vi "Postfix Stack.vi"(8 "error in (no error)":errorcluster, 10 "Variable Names":string[](array[string]), 11 "Postfix":T2[](array[typedef])) -> (0 "error out":errorcluster, 2 "Values":dbl[](array[numeric]), 3 "Types":T1[](array[typedef]))   [LabVIEW 2022 SP3, in "Expressions.lvlib"]
uses:
  Expressions.lvlib
  Controls/Token.ctl
  Controls/Token Type.ctl
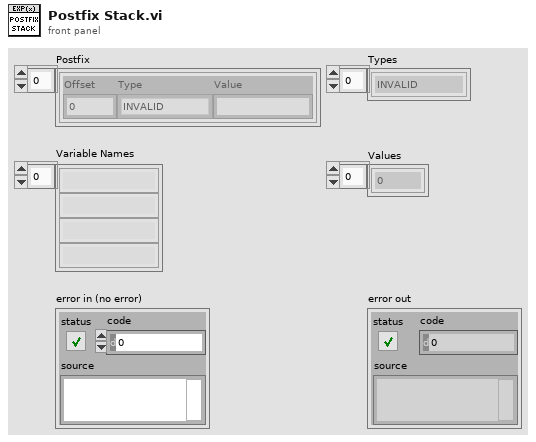
[diagram p1: front panel]
types:
  T1 = typedef "Expressions.lvlib/Token Type.ctl" = enum8{"INVALID", "NOT", "AND", "OR", "EE", "NE", "LT", "GT", "LTE", "GTE", "PLUS", "MINUS", "MULTIPLY", "DIVIDE", "MODULUS", "LPAREN", "RPAREN", "LITERAL", "IDENTIFIER", "DEFINITION"}
  T2 = typedef "Expressions.lvlib/Token.ctl" = cluster{"Offset":i32, "Type":T1, "Value":string}
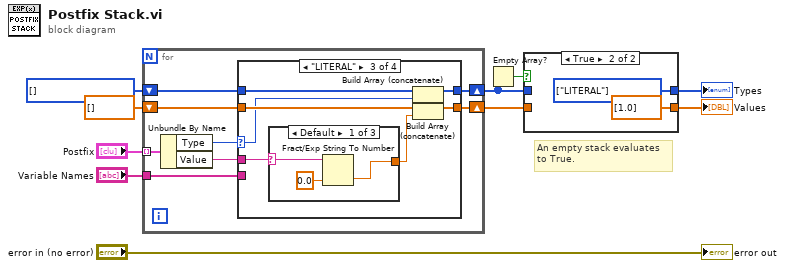
[diagram p0: block diagram]
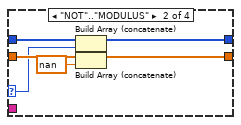
[diagram p4: hidden frame]
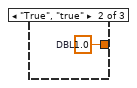
[diagram p5: hidden frame]
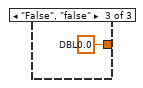
[diagram p6: hidden frame]
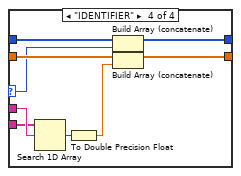
[diagram p7: hidden frame]
diagram:
  w9 = T1[] [] items=["INVALID", "NOT", "AND", "OR", "EE", "NE", "LT", "GT", "LTE", "GTE", "PLUS", "MINUS", "MULTIPLY", "DIVIDE", "MODULUS", "LPAREN", "RPAREN", "LITERAL", "IDENTIFIER", "DEFINITION"]
  # "An empty stack evaluates\nto True."
  n1 = for {
    tunnel: "Postfix" -> [w18] mode=indexing
    shift-right: [w16] -> w7
    shift-left: w9 -> [w15]
    shift-right: [w13] -> w5
    shift-left: dbl[] [] ("Values") -> [w14]
    tunnel: "Variable Names" -> [w11]
    n2 = Unbundle By Name(w18) -> ("Type"=w17:T1, "Value"=w12:string)
    n3 = case shown="\"LITERAL\"" w17 {
      selector: w17 -> [_ w22 w29 w43]
      tunnel: [w20 w24 w31 w45] -> w16
      tunnel: w15 -> [w20 w26 w33 w47]
      tunnel: w14 -> [w19 w25 w32 w46]
      tunnel: [w19 w23 w30 w44] -> w13
      tunnel: w12 -> [_ _ w28 w42]
      tunnel: w11 -> [_ _ _ w41]
      frame "INVALID", "LPAREN", "RPAREN", "DEFINITION" {
      }
      frame "NOT".."MODULUS" {
        n4 = Build Array (concatenate)(w26, w22) -> (w24:T1[])
        n5 = Build Array (concatenate)(w25, nan) -> (w23:dbl[])
      }
      frame "LITERAL" {
        n6 = case shown="Default" w28 {
          selector: w28 -> [w36 _ _]
          tunnel: [w34 w37 w38] -> w27
          frame Default {
            n7 = Fract/Exp String To Number(string=w36, default (0 dbl)=0.0 ("DBL")) -> (number=w34:dbl)  [unwired: 2 in, 1 out]
          }
          frame "True", "true" {
            w37 = 1.0  # DBL
          }
          frame "False", "false" {
            w38 = 0.0  # DBL
          }
        }
        n8 = Build Array (concatenate)(w33, w29) -> (w31:T1[])
        n9 = Build Array (concatenate)(w32, w27) -> (w30:dbl[])
      }
      frame "IDENTIFIER" {
        n10 = Search 1D Array(1D array=w41, element=w42) -> (index of element=w40:i32)  [unwired: 1 in]
        n11 = To Double Precision Float(number=w40) -> (double precision float=w39:dbl)
        n12 = Build Array (concatenate)(w47, w43) -> (w45:T1[])
        n13 = Build Array (concatenate)(w46, w39) -> (w44:dbl[])
      }
    }
  }
  n14 = Empty Array?(array=w7) -> (empty?=w6:bool)
  n15 = case shown="True" w6 {
    tunnel: [w49 w51] -> w2
    tunnel: w7 -> [w49 _]
    tunnel: [w48 dbl[] [1.0] ("Values")] -> w1
    tunnel: w5 -> [w48 _]
    frame False {
    }
    frame True {
      w51 = T1[] [enum."LITERAL"] items=["INVALID", "NOT", "AND", "OR", "EE", "NE", "LT", "GT", "LTE", "GTE", "PLUS", "MINUS", "MULTIPLY", "DIVIDE", "MODULUS", "LPAREN", "RPAREN", "LITERAL", "IDENTIFIER", "DEFINITION"]
    }
  }
  "Types" <- w2
  "Values" <- w1
  "error out" <- "error in (no error)"
